vi "Set Config Value Float.vi"(6 "section":string, 8 "error in (no error)":errorcluster, 9 "value":dbl, 10 "key":string, 11 "Output Actor Hardware Interface":refnum<class "Output Actor Hardware Interface.lvclass">) -> (0 "error out":errorcluster, 3 "Output Actor Hardware Interface out":refnum<class "Output Actor Hardware Interface.lvclass">)   [LabVIEW 2015, in "Output Actor Hardware Interface.lvclass"]
uses:
  Output Actor Hardware Interface.lvclass
  <vilib>/Utility/config.llb/Write Key (Double).vi
  <vilib>/Utility/config.llb/NI_LVConfig.lvlib
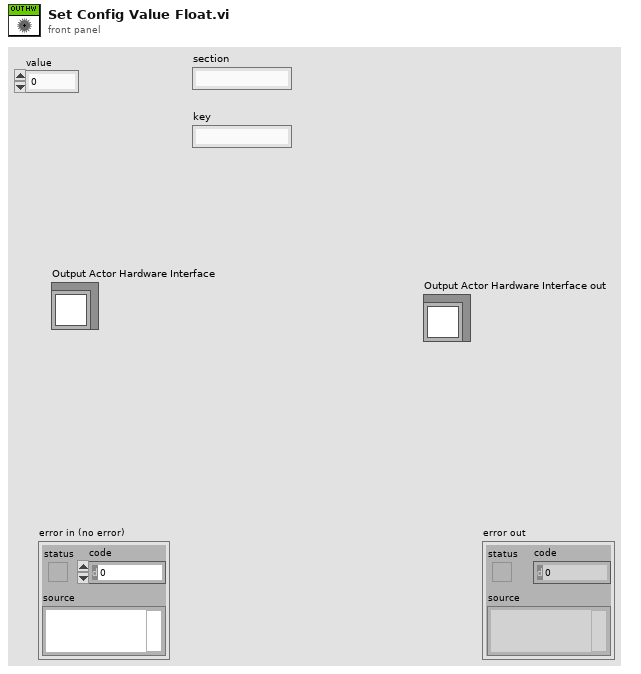
[diagram p1: front panel]
types:
  T1 = typedef "NI_LVConfig.lvlib/Config Data RefNum.ctl" = refnum<k1>
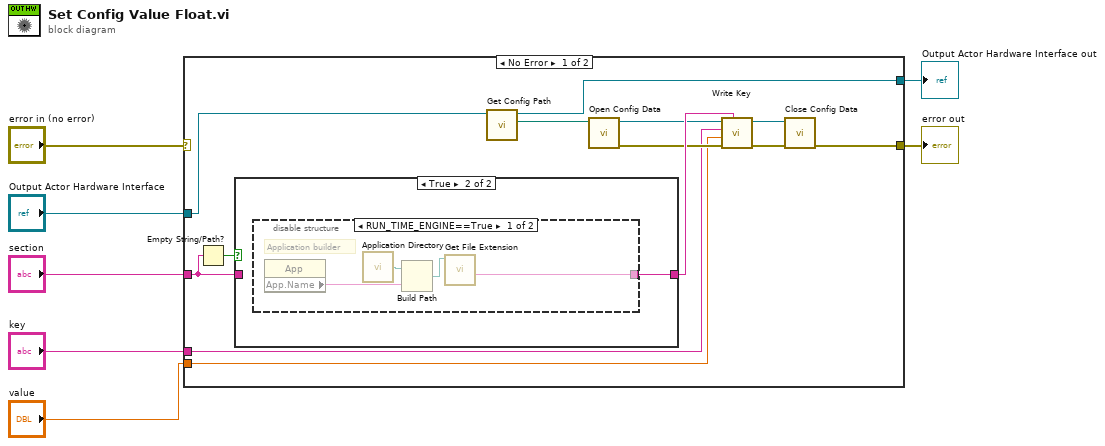
[diagram p0: block diagram]
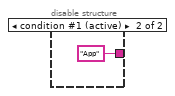
[diagram p3: hidden frame]
diagram:
  n1 = case shown="No Error" "error in (no error)" {
    selector: "error in (no error)" -> [_ w29]
    tunnel: [w13 w29] -> w6
    tunnel: [w12 w28] -> w1
    tunnel: "Output Actor Hardware Interface" -> [w11 w28]
    tunnel: "section" -> [w10 _]
    tunnel: "key" -> [w9 _]
    tunnel: "value" -> [w8 _]
    frame No Error {
      n2 = Empty String/Path?(string/path=w10) -> (empty?=w18:bool)
      n3 = case shown="True" w18 {
        tunnel: [w21 w22] -> w19
        tunnel: w10 -> [w21 _]
        frame False {
        }
        frame True {
          n4 = disable-structure shown="RUN_TIME_ENGINE==True" {
            disable-tunnel: [w23 "App" ("name or relative path")] -> w22
            frame condition #0 {
              # "Application builder"
              n5 = property class="App"() -> ("App.Name"=w26:string)  [unwired: 2 in, 2 out]
              n6 = call <vilib>:"Application Directory.vi"() -> ("Application Directory"=w25:path)
              n7 = Build Path(base path=w25, name or relative path=w26) -> (appended path=w24:path)
              n8 = call <vilib>:"Get File Extension.vi"("file"=w24) -> ("filename without extension"=w23:string)  [unwired: 6 in, 4 out]
            }
            frame condition #1 (active) {
            }
          }
        }
      }
      n9 = call "Get Config Path.vi"("Output Actor Hardware Interface.lvclass"=w11) -> ("Path"=w20:path, "Output Actor Hardware Interface.lvclass 2"=w12:refnum<class "Output Actor Hardware Interface.lvclass">)  [unwired: 9 in]
      n10 = call <vilib>:"Open Config Data.vi"("configuration file path"=w20) -> ("error out"=w16:errorcluster, "refnum"=w14:T1)  [unwired: 8 in, 1 out]
      n11 = call-poly <vilib>:"Write Key.vi"("section"=w19, "error in (no error)"=w16, "value"=w8, "key"=w9, "refnum"=w14) -> ("error out"=w17:errorcluster, "refnum out"=w15:T1)  [unwired: 4 in, 1 out]
      n12 = call <vilib>:"Close Config Data.vi"("error in (no error)"=w17, "refnum"=w15) -> ("error out"=w13:errorcluster)  [unwired: 8 in, 1 out]
    }
    frame Error {
    }
  }
  "error out" <- w6
  "Output Actor Hardware Interface out" <- w1
